vi "Destroy.vi"(8 "Error In":errorcluster, 11 "Session":refnum<class "Session.lvclass">) -> (0 "Error Out":errorcluster, 3 "labssh2 Shared Library":path)   [LabVIEW 2017, in "LabSSH2.lvlib" / "Session.lvclass"]
uses:
  Session.lvclass
  Session.lvclass/Session.ctl
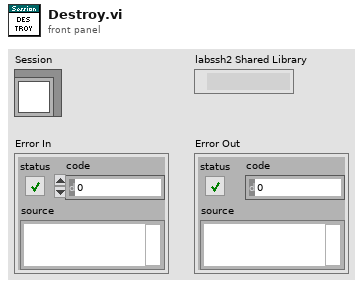
[diagram p1: front panel]
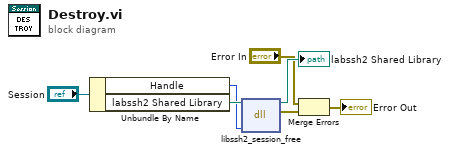
[diagram p0: block diagram]
diagram:
  n1 = Unbundle By Name("Session") -> ("Handle"=w2:u64, "labssh2 Shared Library"=w6:path)
  n2 = dll-call lib="D:/Users/cfield/Code/Field R&D Services/SSH/LabSSH2/LabVIEW/trunk/src/LabSSH2/Private/labssh2.*" fn="libssh2_session_free"(path in=w6, "session"=w2) -> (path out=→"labssh2 Shared Library":path, error out=w1:errorcluster)  [unwired: 4 in]
  n3 = Merge Errors("Error In", w1) -> (→"Error Out":errorcluster)
